vi "Write Consumer Name.vi"(8 "error in (no error)":errorcluster, 10 "Consumer Name":string, 11 "Consumer Name Response Message in":refnum<class "Consumer Name Response Message.lvclass">) -> (0 "error out":errorcluster, 3 "Consumer Name Response Message out":refnum<class "Consumer Name Response Message.lvclass">)   [LabVIEW 2027, in "Consumer Name Response Message.lvclass"]
uses:
  Consumer Name Response Message.lvclass
  Consumer Name Response Message.lvclass/Consumer Name Response Message.ctl
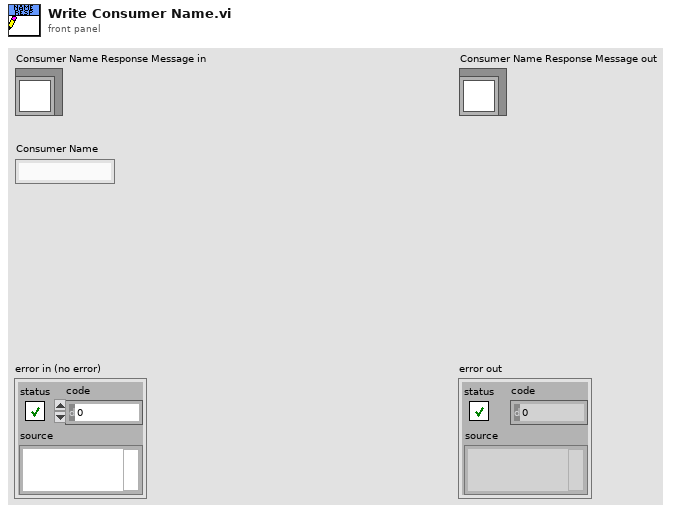
[diagram p1: front panel]
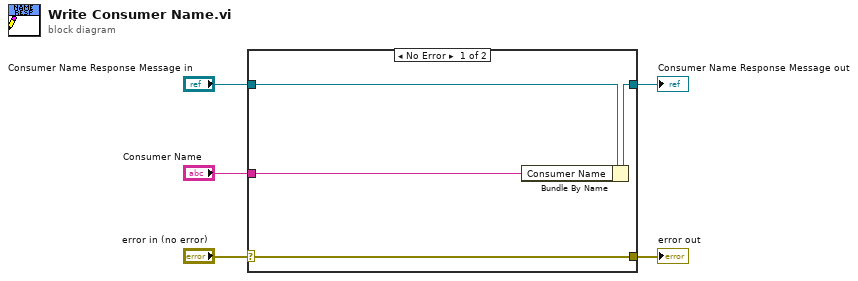
[diagram p0: block diagram]
diagram:
  n1 = case shown="No Error" "error in (no error)" {
    selector: "error in (no error)" -> [w9 w10]
    tunnel: [w9 w10] -> w4
    tunnel: [w7 w11] -> w2
    tunnel: "Consumer Name Response Message in" -> [w8 w11]
    tunnel: "Consumer Name" -> [w6 _]
    frame No Error {
      n2 = Bundle By Name(cluster=w8, "Consumer Name"=w6) -> (w7:refnum<class "Consumer Name Response Message.lvclass">)
    }
    frame Error {
    }
  }
  "error out" <- w4
  "Consumer Name Response Message out" <- w2
